vi "RT Finialize.vi"(8 "error in (no error)":errorcluster, 11 "RT Data Cluster in":T1 {"StatusRefs" format="%.0x"; "ReceiveRefs"."Data Reference" format="%.0x"; "SendRefs"."Data Reference" format="%.0x"}) -> (0 "error out":errorcluster)   [LabVIEW 2012, in "PXImc Engine.lvlib"]
uses:
  PXImc Engine.lvlib
  RT Data Cluster.ctl
  Shared/Compiled Data.ctl
  <vilib>/NI Veristand/Custom Device API/Block Data Reference.ctl
  <vilib>/NI Veristand/Custom Device API/Data Reference.ctl
  <vilib>/pximc/nipximc.lvlib
  Shared/PXImc Shared.lvlib
  <vilib>/NI Veristand/Custom Device API/Custom Device API.lvlib
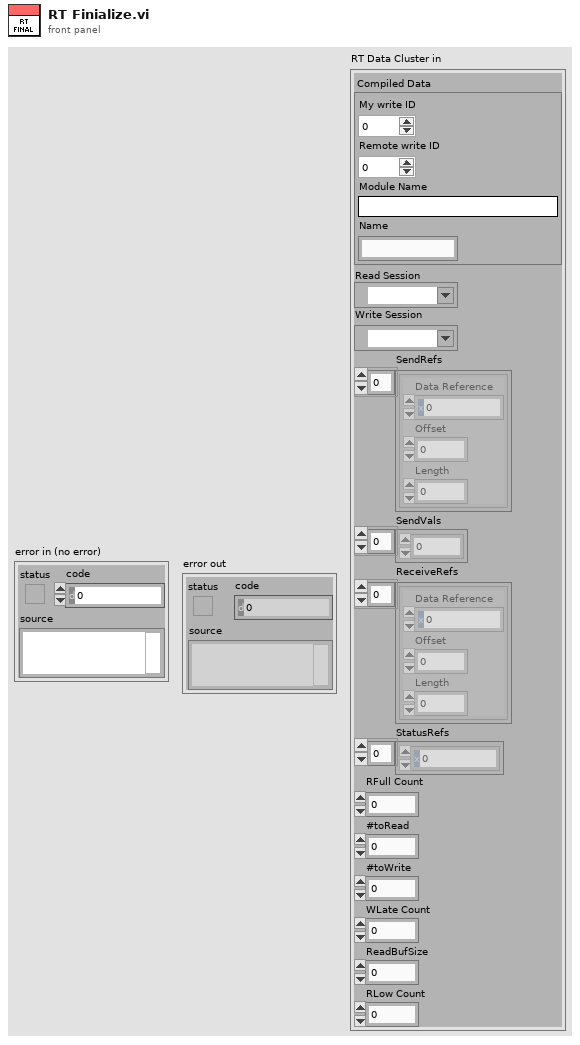
[diagram p1: front panel]
types:
  T1 = typedef "PXImc Engine.lvlib/RT Data Cluster.ctl" = cluster{"Compiled Data":T2, "Read Session":refnum<k21>, "Write Session":refnum<k21>, "SendRefs":T3[], "SendVals":dbl[], "ReceiveRefs":T3[], "StatusRefs":T4[], "RFull Count":dbl, "#toRead":i32, "#toWrite":i32, "WLate Count":dbl, "ReadBufSize":i32, "RLow Count":dbl}
  T2 = typedef "PXImc Shared.lvlib/Compiled Data.ctl" = cluster{"My write ID":u16, "Remote write ID":u16, "Module Name":string, "Name":string}
  T3 = typedef "Custom Device API.lvlib/Block Data Reference.ctl" = cluster{"Data Reference":T4, "Offset":i32, "Length":i32}
  T4 = typedef "Custom Device API.lvlib/Data Reference.ctl" = i32
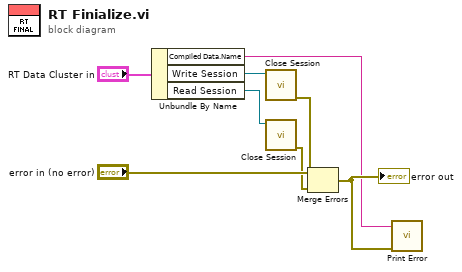
[diagram p0: block diagram]
diagram:
  n1 = Unbundle By Name("RT Data Cluster in") -> ("Compiled Data.Name"=w5:string, "Write Session"=w4:refnum<k21>, "Read Session"=w3:refnum<k21>)
  n2 = call <vilib>:"Close Session.vi"("session in"=w4) -> ("error out"=w2:errorcluster)  [unwired: 10 in]
  n3 = call <vilib>:"Close Session.vi"("session in"=w3) -> ("error out"=w1:errorcluster)  [unwired: 10 in]
  n4 = Merge Errors("error in (no error)", w2, w1) -> (w7:errorcluster)
  "error out" <- w7
  n5 = call "Print Error.vi"("error out"=w7, "Your code's public name"=w5) -> ()  [unwired: 9 in]
